vi "Start Bit.vi"(8 "error in (no error)":errorcluster, 11 "Low Speed in":refnum<class "Low Speed.lvclass">) -> (0 "error out":errorcluster, 3 "Low Speed out":refnum<class "Low Speed.lvclass">)   [LabVIEW 2020, in "Low Speed.lvclass"]
uses:
  Low Speed.lvclass
  C:/Users/kaiser.asan/OneDrive - SolitonTechnologies/LabVIEW/29.SDLC - I2C Driver/I2C Module/I2C Controller Module/Class/Transmission Mode/Parent/TX Speed.lvclass
  Low Speed.lvclass/Low Speed.ctl
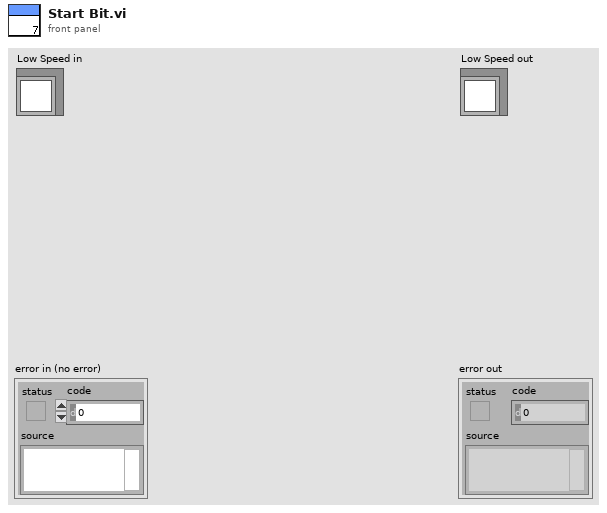
[diagram p1: front panel]
types:
  T1 = typedef "I2C Controller Lib.lvlib/Timing Parameters Cluster.ctl" = cluster{"f_SCL(KHz)":u32, "t_HIGH (ns)":u32, "t_LOW (ns)":u32, "t_SU;STA (ns)":u32, "t_HD;STA (ns)":u32, "t_SU;DAT (ns)":u32, "t_HD;DAT (ns)":u32, "t_SU;STO (ns)":u32, "t_BUF (ns)":u32}
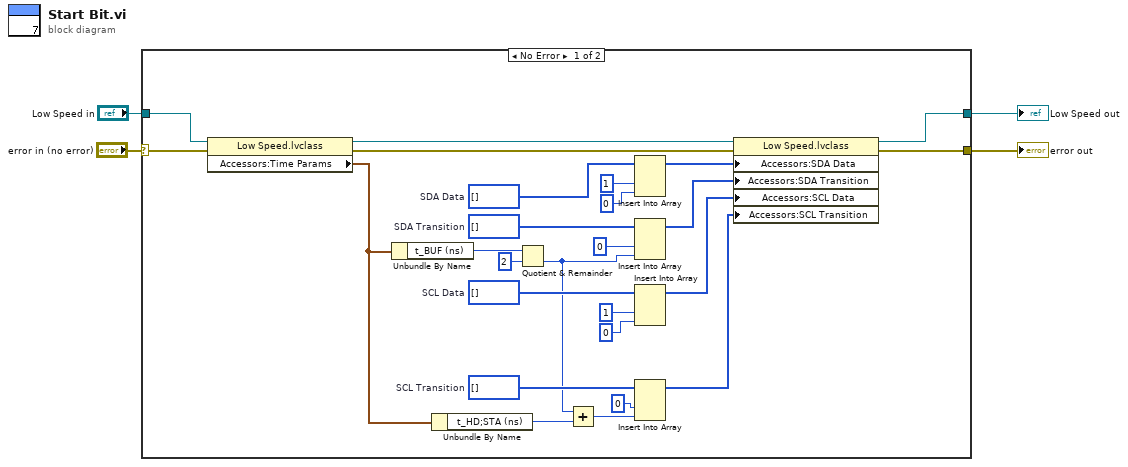
[diagram p0: block diagram]
diagram:
  n1 = case shown="No Error" "error in (no error)" {
    selector: "error in (no error)" -> [w30 w31]
    tunnel: [w20 w31] -> w4
    tunnel: [w18 w32] -> w2
    tunnel: "Low Speed in" -> [w28 w32]
    frame No Error {
      w8 = u8[] []  # SDA Data
      w9 = u32[] []  # SDA Transition
      w10 = u32[] []  # SCL Transition
      w11 = u8[] []  # SCL Data
      n2 = property class="Low Speed.lvclass"(reference=w28, error in=w30) -> (reference out=w19:refnum<class "Low Speed.lvclass">, error out=w29:errorcluster, "Accessors:Time Params"=w13:T1)
      n3 = Unbundle By Name(w13) -> ("t_BUF (ns)"=w23:u32)
      n4 = Unbundle By Name(w13) -> ("t_HD;STA (ns)"=w6:u32)
      n5 = Quotient & Remainder(x=w23, y=u32 2) -> (floor(x/y)=w5:u32)  [unwired: 1 out]
      n6 = Add(x=w5, y=w6) -> (x+y=w7:u32)
      n7 = Insert Into Array(array=w8, new element #1=u8 1 ("new element/subarray"), new element #2=u8 0 ("new element/subarray")) -> (w17:u8[])  [unwired: 1 in]
      n8 = Insert Into Array(array=w9, new element #1=u32 0 ("new element/subarray"), new element #2=w5) -> (w16:u32[])  [unwired: 1 in]
      n9 = Insert Into Array(array=w11, new element #1=u8 1 ("new element/subarray"), new element #2=u8 0 ("new element/subarray")) -> (w15:u8[])  [unwired: 1 in]
      n10 = Insert Into Array(array=w10, new element #1=u32 0 ("new element/subarray"), new element #2=w7) -> (w14:u32[])  [unwired: 1 in]
      n11 = property class="Low Speed.lvclass"(reference=w19, error in=w29, "Accessors:SDA Data"=w17, "Accessors:SDA Transition"=w16, "Accessors:SCL Data"=w15, "Accessors:SCL Transition"=w14) -> (reference out=w18:refnum<class "Low Speed.lvclass">, error out=w20:errorcluster)
    }
    frame Error {
    }
  }
  "error out" <- w4
  "Low Speed out" <- w2
